vi "Xml_Read_Hardware.vi"(8 "error in (no error)":errorcluster, 9 "Version String":string, 10 "XML Path":path=path "D:/TEST.xml", 11 "Variant":variant) -> (0 "error out":errorcluster, 3 "Variant Output":variant)   [LabVIEW 2024]
doc: "This VI reads an XML file of parameters and casts the Resource Name (String) to an IVI Class, as the GXML Lib is unable to read/write objects of type IVI class."
uses:
  <instrlib>/niHSDIO/niHSDIO.llb/niHSDIO_ctl Trigger Source Values (Ring).ctl
  controls/HARDWARE_Inputs.ctl
  controls/AO_6711_Inputs.ctl
  controls/AO_6738_Inputs.ctl
  controls/AWG_5421_Inputs.ctl
  <instrlib>/niFgen/niFgen.llb/niFgen_ctl Trigger Source Values (Ring).ctl
  controls/DIGIT_5122_Inputs.ctl
  <instrlib>/niScope/Controls/niScope trigger source.ctl
  controls/HSDIO_6541_Inputs.ctl
  <vilib>/NI/GXML/_subVIs/GXML SearchParser/Search Parser.vi
  <vilib>/NI/GXML/GXML.lvlib
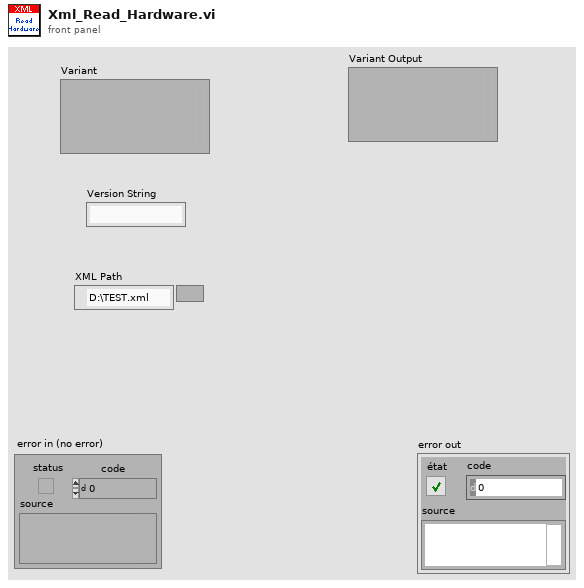
[diagram p1: front panel]
types:
  T1 = typedef "niScope trigger source.ctl" = string
  T2 = cluster{"Sample Rate":dbl, "Resource Name":string, "Channel Name":string, "Trigger Source":T1, "Vertical Range":dbl, "Trigger Level":dbl}
  T3 = typedef "niFgen_ctl Trigger Source Values (Ring).ctl" = string
  T4 = cluster{"Resource Name":string, "Sample Rate":dbl, "Trigger Type":u16, "Trigger Source":T3}
  T5 = typedef "HARDWARE_Inputs.ctl" = cluster{"AO 6711 Inputs":T6, "AO 6738 Inputs":T7, "AWG 5421 Inputs":T8, "DIGIT 5122 Inputs":T9, "HSDIO 6541 Inputs":T10}
  T6 = typedef "AO_6711_Inputs.ctl" = cluster{"Physical Channels":tag, "Min Voltage":dbl, "Max Voltage":dbl, "Trigger Source":tag, "Counter":tag}
  T7 = typedef "AO_6738_Inputs.ctl" = cluster{"Physical Channels":tag, "Min Voltage":dbl, "Max Voltage":dbl, "Trigger Source":tag, "Counter":tag}
  T8 = typedef "AWG_5421_Inputs.ctl" = cluster{"Resource Name":refnum<k15>, "Sample Rate":dbl, "Trigger Type":u16, "Trigger Source":T3, "Waveform Gain":dbl, "Digital Filter ON":bool}
  T9 = typedef "DIGIT_5122_Inputs.ctl" = cluster{"Sample Rate":dbl, "Resource Name":refnum<k15>, "Channel Name":string, "Trigger Source":T1, "Vertical Range":dbl, "Trigger Level":dbl}
  T10 = typedef "HSDIO_6541_Inputs.ctl" = cluster{"Resource Name":refnum<k15>, "Clock Rate":dbl, "Trigger Source":T11}
  T11 = typedef "niHSDIO_ctl Trigger Source Values (Ring).ctl" = string
  T12 = cluster{"Resource Name":string, "Clock Rate":dbl, "Trigger Source":T11}
  T13 = cluster{"Resource Name":string, "Sample Rate":dbl, "Trigger Type":u16, "Trigger Source":T3, "Waveform Gain":dbl, "Digital Filter ON":bool}
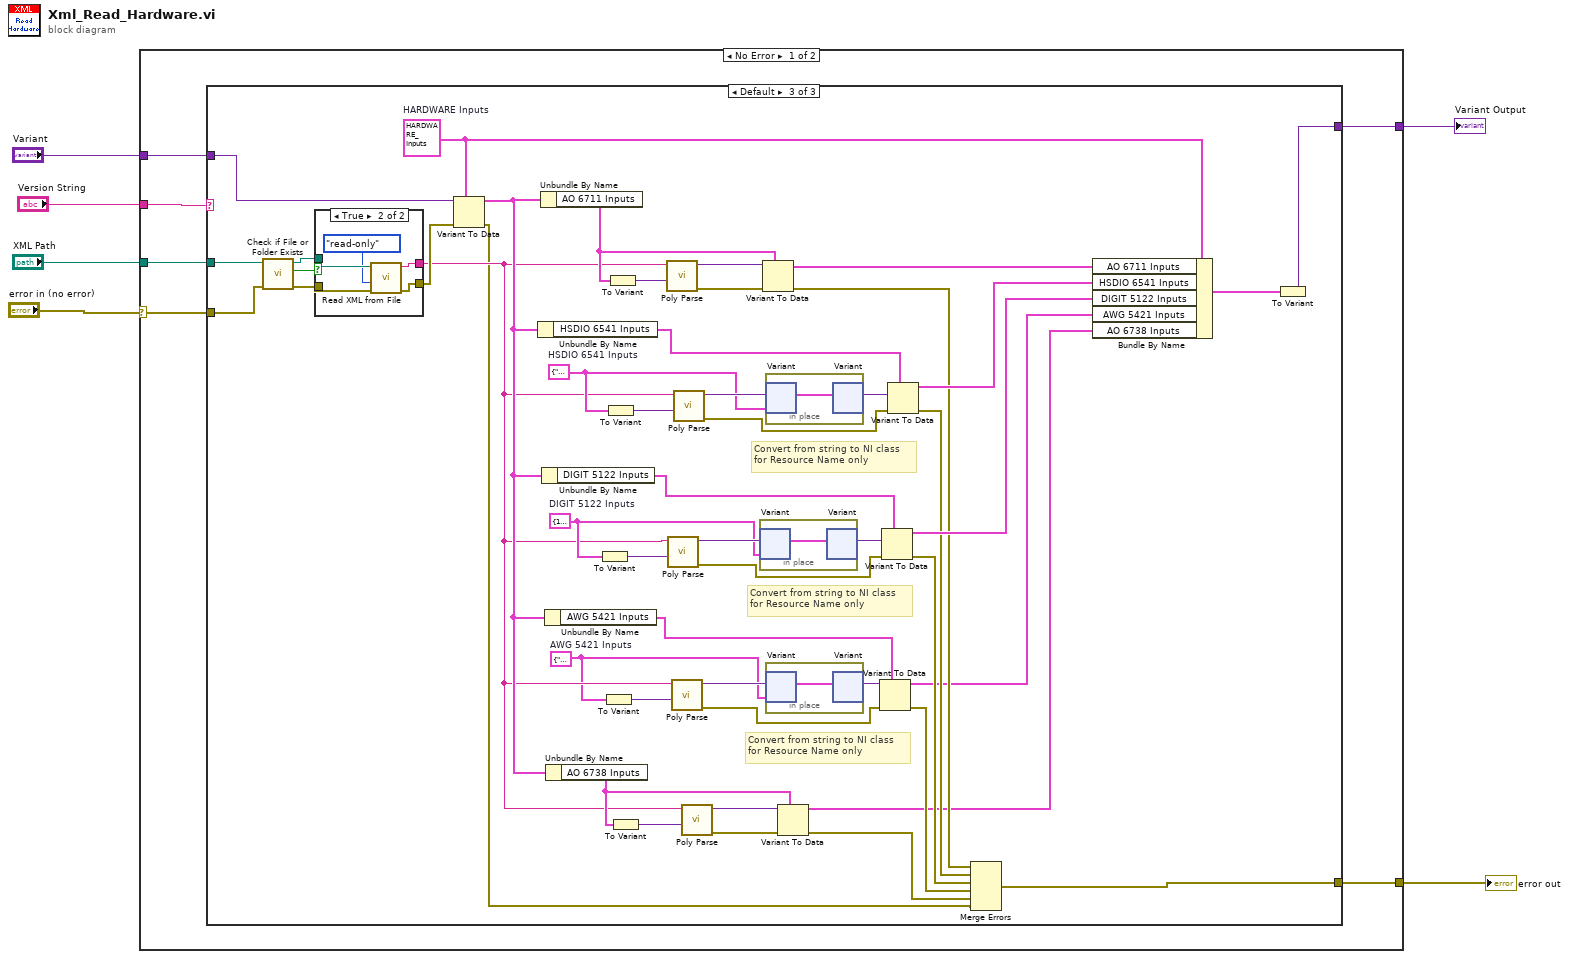
[diagram p0: block diagram]
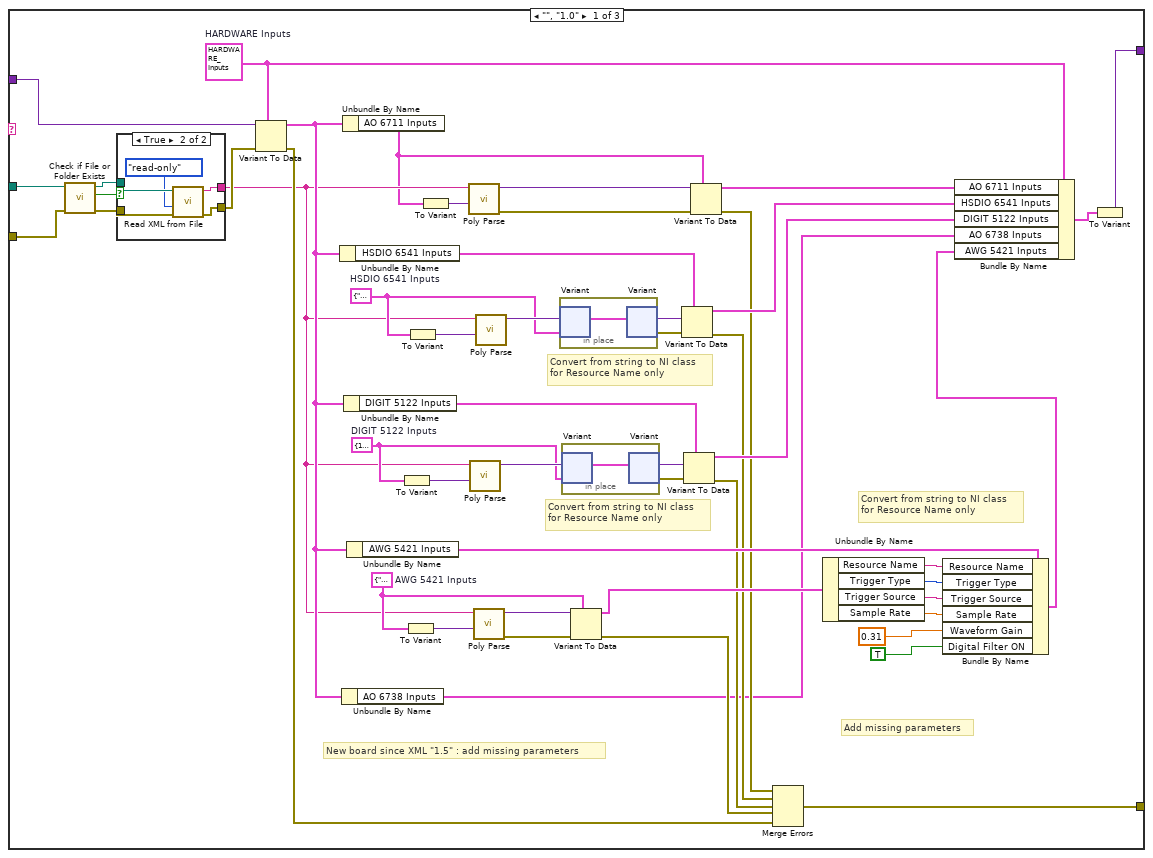
[diagram p2: hidden frame]
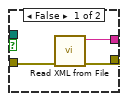
[diagram p3: hidden frame]
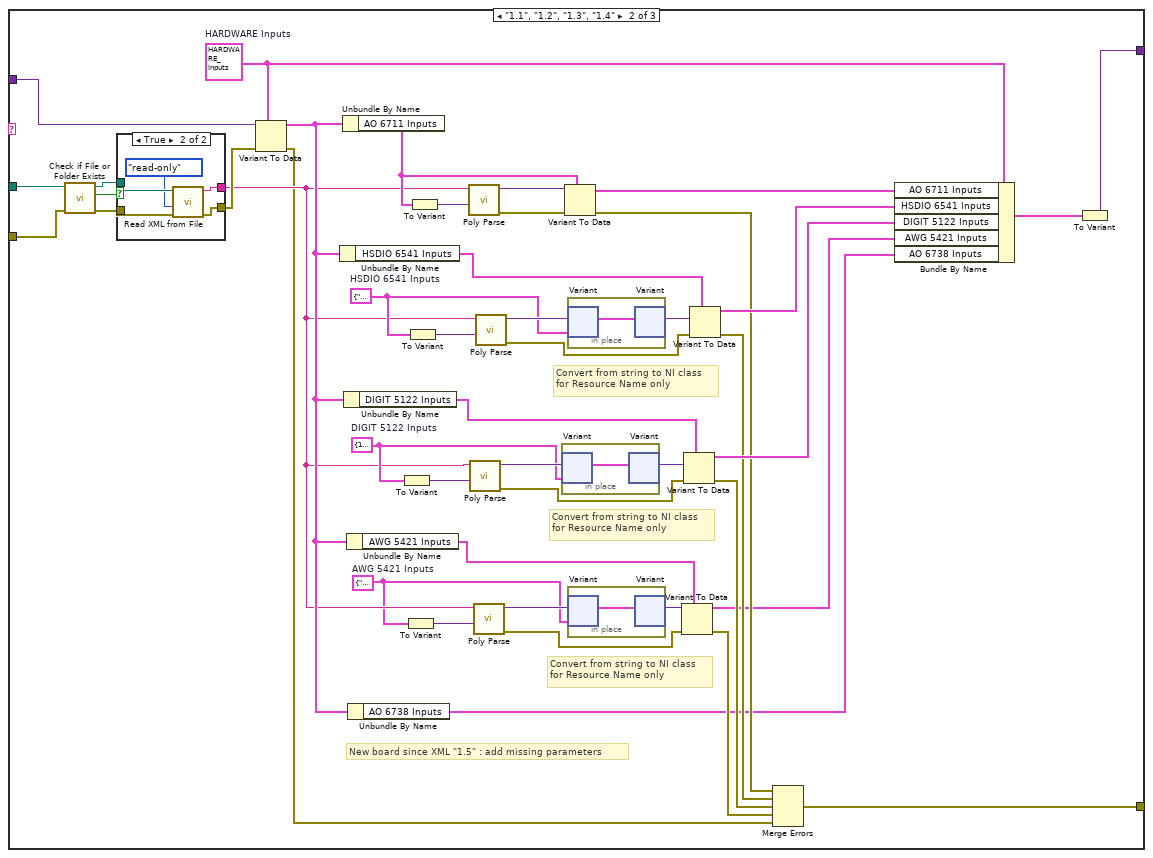
[diagram p4: hidden frame]
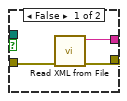
[diagram p5: hidden frame]
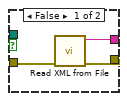
[diagram p6: hidden frame]
diagram:
  n1 = case shown="No Error" "error in (no error)" {
    selector: "error in (no error)" -> [w12 w192]
    tunnel: [w11 w192] -> w5
    tunnel: "XML Path" -> [w10 _]
    tunnel: [w9 w191] -> w3
    tunnel: "Variant" -> [w8 w191]
    tunnel: "Version String" -> [w7 _]
    frame No Error {
      n2 = case shown="Default" w7 {
        tunnel: w12 -> [w60 w115 w176]
        tunnel: [w21 w81 w142] -> w11
        tunnel: w10 -> [w59 w112 w173]
        tunnel: w8 -> [w47 w107 w168]
        tunnel: [w44 w104 w165] -> w9
        frame "", "1.0" {
          w30 = T2 {"Sample Rate"=10000000.0, "Resource Name"="Digitizer", "Channel Name"="0", "Trigger Source"="VAL_EXTERNAL", "Vertical Range"=10.0, "Trigger Level"=3.0}  # DIGIT 5122 Inputs
          w42 = T4 {"Resource Name"="AWG_5421", "Sample Rate"=10000000.0, "Trigger Type"=2, "Trigger Source"="PFI0"}  # AWG 5421 Inputs
          w45 = T5 {"AO 6711 Inputs"={"Physical Channels"="AnalogOutput/ao0:3", "Min Voltage"=-10.0, "Max Voltage"=10.0, "Trigger Source"="/AnalogOutput/PFI0", "Counter"="AnalogOutput/ctr0"}, "AO 6738 Inputs"={"Physical Channels"="AO_6738/ao0:3", "Min Voltage"=-10.0, "Max Voltage"=10.0, "Trigger Source"="/AO_6738/PFI2", "Counter"="AO_6738/ctr0"}, "AWG 5421 Inputs"={"Resource Name"="AnalogOutput/ao0:3", "Sample Rate"=20000000.0, "Trigger Type"=2, "Trigger Source"="PFI0", "Waveform Gain"=0.31, "Digital Filter ON"=TRUE}, "DIGIT 5122 Inputs"={"Sample Rate"=9.0, "Resource Name"="Digitizer", "Channel Name"="PFI0", "Trigger Source"="VAL_EXTERNAL", "Vertical Range"=10.0, "Trigger Level"=3.0}, "HSDIO 6541 Inputs"={"Resource Name"="SequencerHSDIO", "Clock Rate"=1000000.0, "Trigger Source"="PFI0"}}  # HARDWARE Inputs
          w38 = T12 {"Resource Name"="SequencerHSDIO", "Clock Rate"=1000000.0, "Trigger Source"="PFI0"}  # HSDIO 6541 Inputs
          # "New board since XML \"1.5\" : add missing parameters"
          # "Convert from string to NI class\nfor Resource Name only"
          # "Convert from string to NI class\nfor Resource Name only"
          # "Convert from string to NI class\nfor Resource Name only"
          # "Add missing parameters"
          n3 = call <vilib>:"Check if File or Folder Exists.vi"("error in (no error)"=w60, "path"=w59) -> ("error out"=w63:errorcluster, "file or folder exists?"=w62:bool, "dup path"=w61:path)  [unwired: 7 in]
          n4 = case shown="True" w62 {
            tunnel: w61 -> [_ w73]
            tunnel: w63 -> [w68 w71]
            tunnel: [w66 w72] -> w18
            tunnel: [w67 w70] -> w46
            frame False {
              n5 = call <vilib>:"Read XML from File.vi"("error in"=w68) -> ("error out"=w67:errorcluster, "XML String Out"=w66:string)  [unwired: 9 in]
            }
            frame True {
              n6 = call <vilib>:"Read XML from File.vi"("error in"=w71, "file access"=enum16{"read/write", "read-only", "write-only"}."read-only", "XML File Path"=w73) -> ("error out"=w70:errorcluster, "XML String Out"=w72:string)  [unwired: 7 in]
            }
          }
          n7 = Variant To Data(error in=w46, type=w45, Variant=w47) -> (data=w20:T5, error out=w19:errorcluster)
          n8 = Unbundle By Name(w20) -> ("HSDIO 6541 Inputs"=w35:T10)
          n9 = Unbundle By Name(w20) -> ("AO 6738 Inputs"=w16:T7)
          n10 = Unbundle By Name(w20) -> ("AO 6711 Inputs"=w13:T6)
          n11 = Unbundle By Name(w20) -> ("DIGIT 5122 Inputs"=w34:T9)
          n12 = Unbundle By Name(w20) -> ("AWG 5421 Inputs"=w28:T8)
          n13 = To Variant(anything=w30) -> (Variant=w31:variant)
          n14 = To Variant(anything=w42) -> (Variant=w56:variant)
          n15 = To Variant(anything=w38) -> (Variant=w58:variant)
          n16 = To Variant(anything=w13) -> (Variant=w57:variant)
          n17 = call-poly <vilib>:"Poly Parse.vi"("TypeDesc"=w57, "XML String In"=w18) -> ("error out"=w14:errorcluster, "Parsed Data"=w15:variant)  [unwired: 8 in]
          n18 = call-poly <vilib>:"Poly Parse.vi"("TypeDesc"=w31, "XML String In"=w18) -> ("Parsed Data"=w32:variant)  [unwired: 8 in, 1 out]
          n19 = call-poly <vilib>:"Poly Parse.vi"("TypeDesc"=w56, "XML String In"=w18) -> ("error out"=w55:errorcluster, "Parsed Data"=w54:variant)  [unwired: 8 in]
          n20 = call-poly <vilib>:"Poly Parse.vi"("TypeDesc"=w58, "XML String In"=w18) -> ("Parsed Data"=w39:variant)  [unwired: 8 in, 1 out]
          n21 = in-place {
            n22 = in-place-variant #1(w39, w38) -> (w65:T12)  [unwired: 1 out]
            n23 = in-place-variant #1(w65) -> (w37:variant, w26:errorcluster)
          }
          n24 = in-place {
            n25 = in-place-variant #2(w32, w30) -> (w64:T2)  [unwired: 1 out]
            n26 = in-place-variant #2(w64) -> (w33:variant, w27:errorcluster)
          }
          n27 = Variant To Data(error in=w55, type=w42, Variant=w54) -> (data=w50:T4, error out=w25:errorcluster)
          n28 = Variant To Data(error in=w26, type=w35, Variant=w37) -> (data=w36:T10, error out=w23:errorcluster)
          n29 = Variant To Data(error in=w27, type=w34, Variant=w33) -> (data=w29:T9, error out=w24:errorcluster)
          n30 = Variant To Data(error in=w14, type=w13, Variant=w15) -> (data=w48:T6, error out=w22:errorcluster)
          n31 = Merge Errors(w22, w23, w24, w25, w19) -> (w21:errorcluster)
          n32 = Unbundle By Name(w50) -> ("Resource Name"=w51:string, "Trigger Type"=w53:u16, "Trigger Source"=w52:T3, "Sample Rate"=w49:dbl)
          n33 = Bundle By Name(cluster=w28, "Resource Name"=w51, "Trigger Type"=w53, "Trigger Source"=w52, "Sample Rate"=w49, "Waveform Gain"=0.31, "Digital Filter ON"=TRUE) -> (w17:T8)
          n34 = Bundle By Name(cluster=w45, "AO 6711 Inputs"=w48, "HSDIO 6541 Inputs"=w36, "DIGIT 5122 Inputs"=w29, "AO 6738 Inputs"=w16, "AWG 5421 Inputs"=w17) -> (w43:T5)
          n35 = To Variant(anything=w43) -> (Variant=w44:variant)
        }
        frame "1.1", "1.2", "1.3", "1.4" {
          w76 = T13 {"Resource Name"="AWG_5421", "Sample Rate"=10000000.0, "Trigger Type"=2, "Trigger Source"="PFI0", "Waveform Gain"=0.31, "Digital Filter ON"=TRUE}  # AWG 5421 Inputs
          w92 = T2 {"Sample Rate"=10000000.0, "Resource Name"="Digitizer", "Channel Name"="0", "Trigger Source"="VAL_EXTERNAL", "Vertical Range"=10.0, "Trigger Level"=3.0}  # DIGIT 5122 Inputs
          w105 = T5 {"AO 6711 Inputs"={"Physical Channels"="AnalogOutput/ao0:3", "Min Voltage"=-10.0, "Max Voltage"=10.0, "Trigger Source"="/AnalogOutput/PFI0", "Counter"="AnalogOutput/ctr0"}, "AO 6738 Inputs"={"Physical Channels"="AO_6738/ao0:3", "Min Voltage"=-10.0, "Max Voltage"=10.0, "Trigger Source"="/AO_6738/PFI2", "Counter"="AO_6738/ctr0"}, "AWG 5421 Inputs"={"Resource Name"="AnalogOutput/ao0:3", "Sample Rate"=20000000.0, "Trigger Type"=2, "Trigger Source"="PFI0", "Waveform Gain"=0.31, "Digital Filter ON"=TRUE}, "DIGIT 5122 Inputs"={"Sample Rate"=9.0, "Resource Name"="Digitizer", "Channel Name"="PFI0", "Trigger Source"="VAL_EXTERNAL", "Vertical Range"=10.0, "Trigger Level"=3.0}, "HSDIO 6541 Inputs"={"Resource Name"="SequencerHSDIO", "Clock Rate"=1000000.0, "Trigger Source"="PFI0"}}  # HARDWARE Inputs
          w100 = T12 {"Resource Name"="SequencerHSDIO", "Clock Rate"=1000000.0, "Trigger Source"="PFI0"}  # HSDIO 6541 Inputs
          # "New board since XML \"1.5\" : add missing parameters"
          # "Convert from string to NI class\nfor Resource Name only"
          # "Convert from string to NI class\nfor Resource Name only"
          # "Convert from string to NI class\nfor Resource Name only"
          n36 = call <vilib>:"Check if File or Folder Exists.vi"("error in (no error)"=w115, "path"=w112) -> ("error out"=w118:errorcluster, "file or folder exists?"=w117:bool, "dup path"=w116:path)  [unwired: 7 in]
          n37 = case shown="True" w117 {
            tunnel: w116 -> [_ w129]
            tunnel: w118 -> [w124 w127]
            tunnel: [w122 w128] -> w79
            tunnel: [w123 w126] -> w106
            frame False {
              n38 = call <vilib>:"Read XML from File.vi"("error in"=w124) -> ("error out"=w123:errorcluster, "XML String Out"=w122:string)  [unwired: 9 in]
            }
            frame True {
              n39 = call <vilib>:"Read XML from File.vi"("error in"=w127, "file access"=enum16{"read/write", "read-only", "write-only"}."read-only", "XML File Path"=w129) -> ("error out"=w126:errorcluster, "XML String Out"=w128:string)  [unwired: 7 in]
            }
          }
          n40 = Variant To Data(error in=w106, type=w105, Variant=w107) -> (data=w80:T5, error out=w78:errorcluster)
          n41 = Unbundle By Name(w80) -> ("HSDIO 6541 Inputs"=w97:T10)
          n42 = Unbundle By Name(w80) -> ("AO 6711 Inputs"=w102:T6)
          n43 = Unbundle By Name(w80) -> ("DIGIT 5122 Inputs"=w96:T9)
          n44 = Unbundle By Name(w80) -> ("AWG 5421 Inputs"=w87:T8)
          n45 = Unbundle By Name(w80) -> ("AO 6738 Inputs"=w74:T7)
          n46 = To Variant(anything=w92) -> (Variant=w93:variant)
          n47 = To Variant(anything=w76) -> (Variant=w109:variant)
          n48 = To Variant(anything=w100) -> (Variant=w111:variant)
          n49 = To Variant(anything=w102) -> (Variant=w110:variant)
          n50 = call-poly <vilib>:"Poly Parse.vi"("TypeDesc"=w110, "XML String In"=w79) -> ("error out"=w113:errorcluster, "Parsed Data"=w114:variant)  [unwired: 8 in]
          n51 = call-poly <vilib>:"Poly Parse.vi"("TypeDesc"=w93, "XML String In"=w79) -> ("error out"=w83:errorcluster, "Parsed Data"=w94:variant)  [unwired: 8 in]
          n52 = call-poly <vilib>:"Poly Parse.vi"("TypeDesc"=w109, "XML String In"=w79) -> ("error out"=w82:errorcluster, "Parsed Data"=w77:variant)  [unwired: 8 in]
          n53 = call-poly <vilib>:"Poly Parse.vi"("TypeDesc"=w111, "XML String In"=w79) -> ("error out"=w84:errorcluster, "Parsed Data"=w101:variant)  [unwired: 8 in]
          n54 = in-place {
            n55 = in-place-variant #3(w94, w92) -> (w120:T2)  [unwired: 1 out]
            n56 = in-place-variant #3(w120) -> (w95:variant)  [unwired: 1 out]
          }
          n57 = Variant To Data(error in=w113, type=w102, Variant=w114) -> (data=w108:T6, error out=w88:errorcluster)
          n58 = in-place {
            n59 = in-place-variant #4(w101, w100) -> (w121:T12)  [unwired: 1 out]
            n60 = in-place-variant #4(w121) -> (w99:variant)  [unwired: 1 out]
          }
          n61 = in-place {
            n62 = in-place-variant #5(w77, w76) -> (w119:T13)  [unwired: 1 out]
            n63 = in-place-variant #5(w119) -> (w75:variant)  [unwired: 1 out]
          }
          n64 = Variant To Data(error in=w82, type=w87, Variant=w75) -> (data=w86:T8, error out=w85:errorcluster)
          n65 = Variant To Data(error in=w83, type=w96, Variant=w95) -> (data=w91:T9, error out=w90:errorcluster)
          n66 = Variant To Data(error in=w84, type=w97, Variant=w99) -> (data=w98:T10, error out=w89:errorcluster)
          n67 = Merge Errors(w88, w89, w90, w85, w78) -> (w81:errorcluster)
          n68 = Bundle By Name(cluster=w105, "AO 6711 Inputs"=w108, "HSDIO 6541 Inputs"=w98, "DIGIT 5122 Inputs"=w91, "AWG 5421 Inputs"=w86, "AO 6738 Inputs"=w74) -> (w103:T5)
          n69 = To Variant(anything=w103) -> (Variant=w104:variant)
        }
        frame Default {
          w131 = T13 {"Resource Name"="AWG_5421", "Sample Rate"=10000000.0, "Trigger Type"=2, "Trigger Source"="PFI0", "Waveform Gain"=0.31, "Digital Filter ON"=TRUE}  # AWG 5421 Inputs
          w153 = T2 {"Sample Rate"=10000000.0, "Resource Name"="Digitizer", "Channel Name"="0", "Trigger Source"="VAL_EXTERNAL", "Vertical Range"=10.0, "Trigger Level"=3.0}  # DIGIT 5122 Inputs
          w166 = T5 {"AO 6711 Inputs"={"Physical Channels"="AnalogOutput/ao0:3", "Min Voltage"=-10.0, "Max Voltage"=10.0, "Trigger Source"="/AnalogOutput/PFI0", "Counter"="AnalogOutput/ctr0"}, "AO 6738 Inputs"={"Physical Channels"="AO_6738/ao0:3", "Min Voltage"=-10.0, "Max Voltage"=10.0, "Trigger Source"="/AO_6738/PFI2", "Counter"="AO_6738/ctr0"}, "AWG 5421 Inputs"={"Resource Name"="AnalogOutput/ao0:3", "Sample Rate"=20000000.0, "Trigger Type"=2, "Trigger Source"="PFI0", "Waveform Gain"=0.31, "Digital Filter ON"=TRUE}, "DIGIT 5122 Inputs"={"Sample Rate"=9.0, "Resource Name"="Digitizer", "Channel Name"="PFI0", "Trigger Source"="VAL_EXTERNAL", "Vertical Range"=10.0, "Trigger Level"=3.0}, "HSDIO 6541 Inputs"={"Resource Name"="SequencerHSDIO", "Clock Rate"=1000000.0, "Trigger Source"="PFI0"}}  # HARDWARE Inputs
          w161 = T12 {"Resource Name"="SequencerHSDIO", "Clock Rate"=1000000.0, "Trigger Source"="PFI0"}  # HSDIO 6541 Inputs
          # "Convert from string to NI class\nfor Resource Name only"
          # "Convert from string to NI class\nfor Resource Name only"
          # "Convert from string to NI class\nfor Resource Name only"
          n70 = call <vilib>:"Check if File or Folder Exists.vi"("error in (no error)"=w176, "path"=w173) -> ("error out"=w179:errorcluster, "file or folder exists?"=w178:bool, "dup path"=w177:path)  [unwired: 7 in]
          n71 = case shown="True" w178 {
            tunnel: w177 -> [_ w190]
            tunnel: w179 -> [w185 w188]
            tunnel: [w183 w189] -> w136
            tunnel: [w184 w187] -> w167
            frame False {
              n72 = call <vilib>:"Read XML from File.vi"("error in"=w185) -> ("error out"=w184:errorcluster, "XML String Out"=w183:string)  [unwired: 9 in]
            }
            frame True {
              n73 = call <vilib>:"Read XML from File.vi"("error in"=w188, "file access"=enum16{"read/write", "read-only", "write-only"}."read-only", "XML File Path"=w190) -> ("error out"=w187:errorcluster, "XML String Out"=w189:string)  [unwired: 7 in]
            }
          }
          n74 = Variant To Data(error in=w167, type=w166, Variant=w168) -> (data=w137:T5, error out=w133:errorcluster)
          n75 = Unbundle By Name(w137) -> ("HSDIO 6541 Inputs"=w158:T10)
          n76 = Unbundle By Name(w137) -> ("AO 6711 Inputs"=w163:T6)
          n77 = Unbundle By Name(w137) -> ("DIGIT 5122 Inputs"=w157:T9)
          n78 = Unbundle By Name(w137) -> ("AWG 5421 Inputs"=w148:T8)
          n79 = Unbundle By Name(w137) -> ("AO 6738 Inputs"=w138:T7)
          n80 = To Variant(anything=w153) -> (Variant=w154:variant)
          n81 = To Variant(anything=w131) -> (Variant=w170:variant)
          n82 = To Variant(anything=w161) -> (Variant=w172:variant)
          n83 = To Variant(anything=w163) -> (Variant=w171:variant)
          n84 = To Variant(anything=w138) -> (Variant=w141:variant)
          n85 = call-poly <vilib>:"Poly Parse.vi"("TypeDesc"=w171, "XML String In"=w136) -> ("error out"=w174:errorcluster, "Parsed Data"=w175:variant)  [unwired: 8 in]
          n86 = call-poly <vilib>:"Poly Parse.vi"("TypeDesc"=w154, "XML String In"=w136) -> ("error out"=w144:errorcluster, "Parsed Data"=w155:variant)  [unwired: 8 in]
          n87 = call-poly <vilib>:"Poly Parse.vi"("TypeDesc"=w170, "XML String In"=w136) -> ("error out"=w143:errorcluster, "Parsed Data"=w132:variant)  [unwired: 8 in]
          n88 = call-poly <vilib>:"Poly Parse.vi"("TypeDesc"=w172, "XML String In"=w136) -> ("error out"=w145:errorcluster, "Parsed Data"=w162:variant)  [unwired: 8 in]
          n89 = call-poly <vilib>:"Poly Parse.vi"("TypeDesc"=w141, "XML String In"=w136) -> ("error out"=w140:errorcluster, "Parsed Data"=w139:variant)  [unwired: 8 in]
          n90 = in-place {
            n91 = in-place-variant #6(w155, w153) -> (w181:T2)  [unwired: 1 out]
            n92 = in-place-variant #6(w181) -> (w156:variant)  [unwired: 1 out]
          }
          n93 = Variant To Data(error in=w174, type=w163, Variant=w175) -> (data=w169:T6, error out=w149:errorcluster)
          n94 = in-place {
            n95 = in-place-variant #7(w162, w161) -> (w182:T12)  [unwired: 1 out]
            n96 = in-place-variant #7(w182) -> (w160:variant)  [unwired: 1 out]
          }
          n97 = in-place {
            n98 = in-place-variant #8(w132, w131) -> (w180:T13)  [unwired: 1 out]
            n99 = in-place-variant #8(w180) -> (w130:variant)  [unwired: 1 out]
          }
          n100 = Variant To Data(error in=w140, type=w138, Variant=w139) -> (data=w135:T7, error out=w134:errorcluster)
          n101 = Variant To Data(error in=w143, type=w148, Variant=w130) -> (data=w147:T8, error out=w146:errorcluster)
          n102 = Variant To Data(error in=w144, type=w157, Variant=w156) -> (data=w152:T9, error out=w151:errorcluster)
          n103 = Variant To Data(error in=w145, type=w158, Variant=w160) -> (data=w159:T10, error out=w150:errorcluster)
          n104 = Merge Errors(w149, w150, w151, w146, w134, w133) -> (w142:errorcluster)
          n105 = Bundle By Name(cluster=w166, "AO 6711 Inputs"=w169, "HSDIO 6541 Inputs"=w159, "DIGIT 5122 Inputs"=w152, "AWG 5421 Inputs"=w147, "AO 6738 Inputs"=w135) -> (w164:T5)
          n106 = To Variant(anything=w164) -> (Variant=w165:variant)
        }
      }
    }
    frame Error {
    }
  }
  "error out" <- w5
  "Variant Output" <- w3
